vi "Initialize.vi"(8 "error in (no error)":errorcluster, 11 "VICI Settings":T1) -> (0 "error out":errorcluster, 1 "Initialized":bool, 2 "No Pump Connected":bool, 3 "VICI Settings":T1)   [LabVIEW 2018, in "VICI M6 M50 Party Mode.lvlib"]
uses:
  VICI M6 M50 Party Mode.lvlib
  Settings Cluster.ctl
  <vilib>/Instr/_visa.llb/VISA Configure Serial Port (Instr).vi
panel:
  out "Bytes at Port 2":u32
  out "Bytes at Port":u32
  out "read buffer 5":string
  out "read buffer 4":string
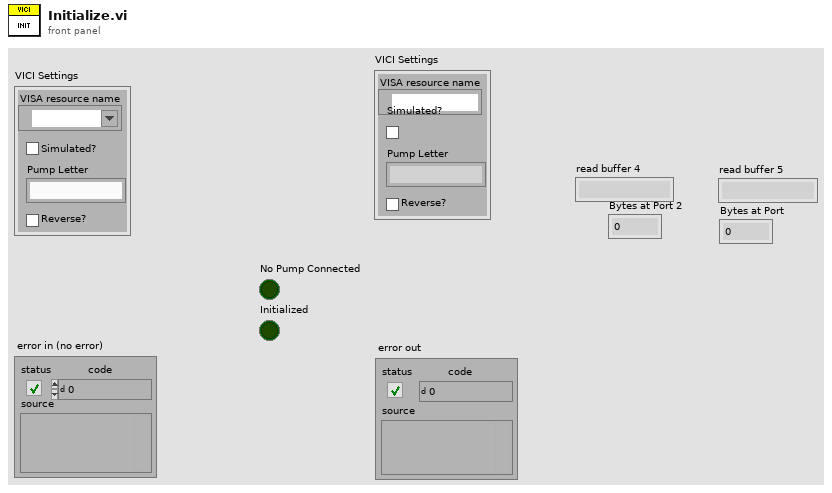
[diagram p1: front panel]
types:
  T1 = typedef "VICI M6 M50 Party Mode.lvlib/Settings Cluster.ctl" = cluster{"VISA resource name":refnum<visa-resource-name>, "Simulated?":bool, "Pump Letter":string, "Reverse?":bool}
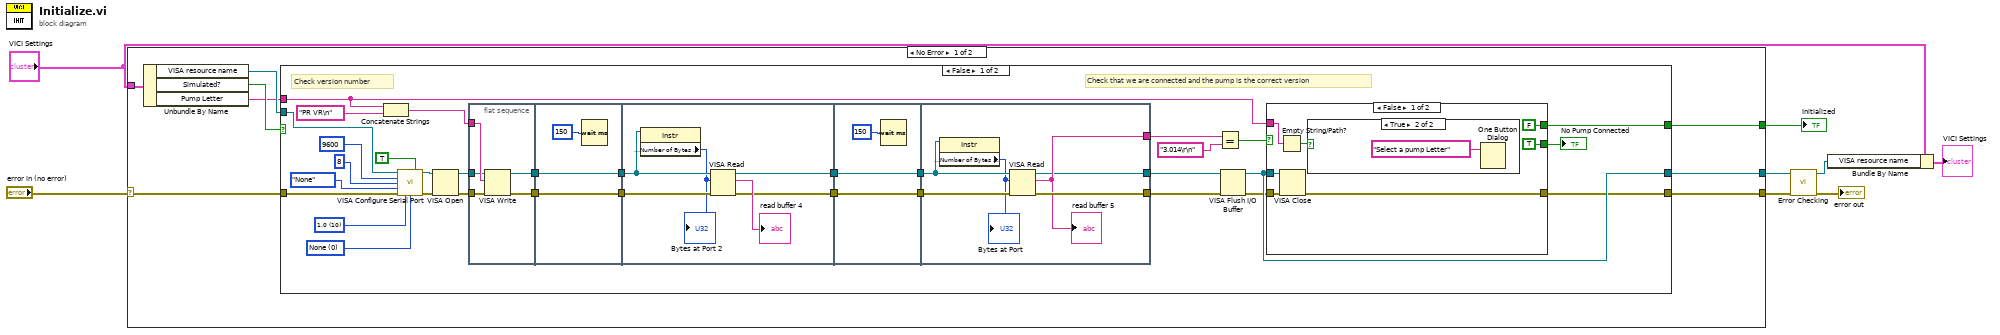
[diagram p0: block diagram]
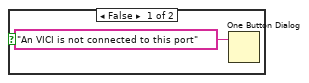
[diagram p2: hidden frame]
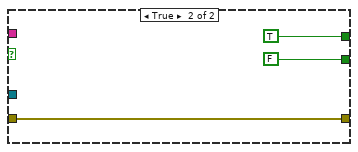
[diagram p3: hidden frame]
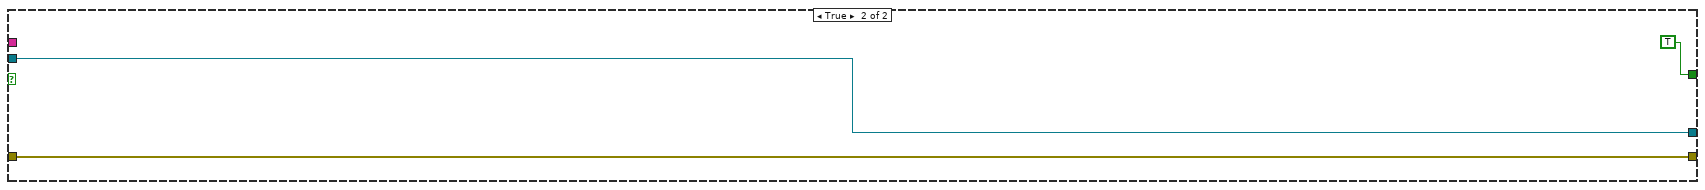
[diagram p4: hidden frame]
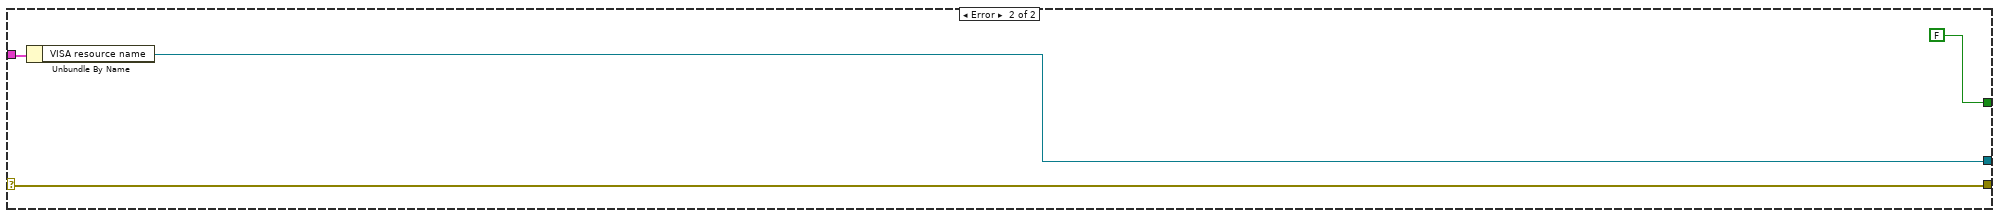
[diagram p5: hidden frame]
diagram:
  n1 = case shown="No Error" "error in (no error)" {
    selector: "error in (no error)" -> [w16 w91]
    tunnel: "VICI Settings" -> [w13 w90]
    tunnel: [w14 w91] -> w4
    tunnel: [w11 w89] -> w5
    tunnel: [w9 FALSE] -> w1
    frame No Error {
      n2 = Unbundle By Name(w13) -> ("VISA resource name"=w12:refnum<visa-resource-name>, "Simulated?"=w15:bool, "Pump Letter"=w10:string)
      n3 = case shown="False" w15 {
        tunnel: w16 -> [w43 w87]
        tunnel: [w27 w87] -> w14
        tunnel: [w31 w86] -> w11
        tunnel: w12 -> [w41 w86]
        tunnel: w10 -> [w23 _]
        tunnel: [w26 TRUE] -> w9
        frame False {
          w45 = u16 0 items=["None", "XON/XOFF", "RTS/CTS", "XON/XOFF & RTS/CTS", "DTR/DSR", "XON/XOFF & DTR/DSR"] ("flow control (0:none)")
          w46 = u16 10 items=["1.0"=10, "1.5"=15, "2.0"=20] ("stop bits (10: 1 bit)")
          # "Check version number"
          # "Check that we are connected and the pump is the correct version"
          n4 = Concatenate Strings(w23, "PR VR\n" ("string")) -> (w24:string)
          n5 = call-poly "VISA Configure Serial Port"("VISA resource name"=w41, "Enable Termination\nChar (T)"=TRUE ("Enable Termination\nChar (T)"), "baud rate (9600)"=u32 9600, "data bits (8)"=u16 8, "parity (0:none)"=enum16{"None", "Odd", "Even", "Mark", "Space"}."None", "error in (no error)"=w43, "stop bits (10: 1 bit)"=w46, "flow control (0:none)"=w45) -> ("VISA resource name out"=w42:refnum<visa-resource-name>, "error out"=w44:errorcluster)  [unwired: 6 in]
          n6 = VISA Open(error in (no error)=w44, VISA resource name=w42) -> (VISA resource name=w18:refnum<visa-resource-name>, error out=w17:errorcluster)  [unwired: 3 in]
          n7 = flat-sequence {
            tunnel: w24 -> [w54]
            tunnel: [w53] -> w36
            tunnel: [w52] -> w35
            tunnel: w18 -> [w51]
            tunnel: w17 -> [w50]
            tunnel: [w55] -> w37
            tunnel: w36 -> [w55]
            tunnel: w35 -> [w56]
            tunnel: [w56] -> w34
            tunnel: w37 -> [w59]
            tunnel: w34 -> [w63]
            tunnel: [w61] -> w22
            tunnel: [w60] -> w20
            tunnel: w22 -> [w66]
            tunnel: [w66] -> w21
            tunnel: w20 -> [w65]
            tunnel: [w65] -> w19
            tunnel: w21 -> [w72]
            tunnel: w19 -> [w68]
            tunnel: [w71] -> w32
            tunnel: [w70] -> w38
            tunnel: [w69] -> w33
            frame #0 {
              n8 = VISA Write(VISA resource name=w51, write buffer=w54, error in (no error)=w50) -> (VISA resource name out=w53:refnum<visa-resource-name>, error out=w52:errorcluster)  [unwired: 1 out]
            }
            frame #1 {
              n9 = Wait (ms)(milliseconds to wait=u32 150) -> ()  [unwired: 1 out]
            }
            frame #2 {
              n10 = property class="Instr"(reference=w59) -> ("Serial Settings:Number of Bytes at Serial Port"=w58:u32)  [unwired: 1 in, 2 out]
              "Bytes at Port 2" <- w58
              n11 = VISA Read(VISA resource name=w59, byte count=w58, error in (no error)=w63) -> (VISA resource name out=w60:refnum<visa-resource-name>, read buffer=→"read buffer 4":string, error out=w61:errorcluster)  [unwired: 1 out]
            }
            frame #3 {
              n12 = Wait (ms)(milliseconds to wait=u32 150) -> ()  [unwired: 1 out]
            }
            frame #4 {
              n13 = property class="Instr"(reference=w68) -> ("Serial Settings:Number of Bytes at Serial Port"=w67:u32)  [unwired: 1 in, 2 out]
              "Bytes at Port" <- w67
              n14 = VISA Read(VISA resource name=w68, byte count=w67, error in (no error)=w72) -> (VISA resource name out=w69:refnum<visa-resource-name>, read buffer=w70:string, error out=w71:errorcluster)  [unwired: 1 out]
              "read buffer 5" <- w70
            }
          }
          n15 = Equal?(x=w38, y="3.014\r\n") -> (x = y?=w39:bool)
          n16 = VISA Flush I/O Buffer(VISA resource name=w33, error in (no error)=w32) -> (VISA resource name out=w31:refnum<visa-resource-name>, error out=w28:errorcluster)  [unwired: 1 in]
          n17 = case shown="False" w39 {
            tunnel: w31 -> [w79 _]
            tunnel: w28 -> [w78 w82]
            tunnel: [TRUE FALSE] -> w29
            tunnel: [w76 w82] -> w27
            tunnel: [FALSE TRUE] -> w26
            tunnel: w23 -> [w73 _]
            frame False {
              n18 = Empty String/Path?(string/path=w73) -> (empty?=w74:bool)
              n19 = VISA Close(VISA resource name=w79, error in (no error)=w78) -> (error out=w76:errorcluster)
              n20 = case shown="True" w74 {
                frame False {
                  n21 = One Button Dialog(message="An VICI is not connected to this port") -> ()  [unwired: 1 in, 1 out]
                }
                frame True {
                  n22 = One Button Dialog(message="Select a pump Letter") -> ()  [unwired: 1 in, 1 out]
                }
              }
            }
            frame True {
            }
          }
          "No Pump Connected" <- w29
        }
        frame True {
        }
      }
    }
    frame Error {
      n23 = Unbundle By Name(w90) -> ("VISA resource name"=w89:refnum<visa-resource-name>)
    }
  }
  "Initialized" <- w1
  n24 = call "Error Checking.vi"("error in (no error)"=w4, "VISA resource name"=w5) -> ("error out"=→"error out":errorcluster, "VISA resource name"=w2:refnum<visa-resource-name>)  [unwired: 7 in, 1 out]
  n25 = Bundle By Name(cluster="VICI Settings", "VISA resource name"=w2) -> (→"VICI Settings":T1)
